vi "LJstreamUD write config.vi"(0 "Working Directory":path, 1 "Data File Prefix":string="data", 2 "Scan Rate (Hz)":dbl=500.0 format="%.3f", 3 "Graph History":i32=1000 min=0, 4 "# Channels":i32=4, 5 "filename":string="ljstreamud.cfg", 6 "Disable Scaling":bool, 7 "Max File Size (Bytes)":i32=1048576, 9 "Write To File":bool, 10 "Channel Setup":T1={"+Ch"=["0", "1", "2", "3", "4", "5", "6", "7"], "-Ch"=["199", "199", "199", "199", "199", "199", "199", "199"], "Ranges"=[0, 0, 0, 0, 0, 0, 0, 0], "Scaling Equation"=["y=v0", "y=v1", "y=v2", "y=v3", "y=v4", "y=v5", "y=v6", "y=v7"], "Graph?"=[]} {"Ranges" items=["LJ_rgBIP10V", "LJ_rgBIP5V", "LJ_rgUNI5V", "LJ_rgUNI2P5V", "LJ_rgUNI1P25V", "LJ_rgBIP1V", "LJ_rgUNIP625V", "LJ_rgBIPP1V", "LJ_rgBIPP01V"]}, 12 "Interval (ms)":u32=500, 13 "Resolution":u8, 14 "SettlingFactor":u8) -> (15 "error out":errorcluster)   [LabVIEW 2021]
uses:
  <vilib>/Utility/config.llb/Write Key (String).vi
  <vilib>/Utility/config.llb/Write Key (U32).vi
  <vilib>/Utility/config.llb/Write Key (Double).vi
  <vilib>/Utility/config.llb/Write Key (I32).vi
  <vilib>/Utility/config.llb/Write Key (Boolean).vi
  <vilib>/Utility/config.llb/NI_LVConfig.lvlib
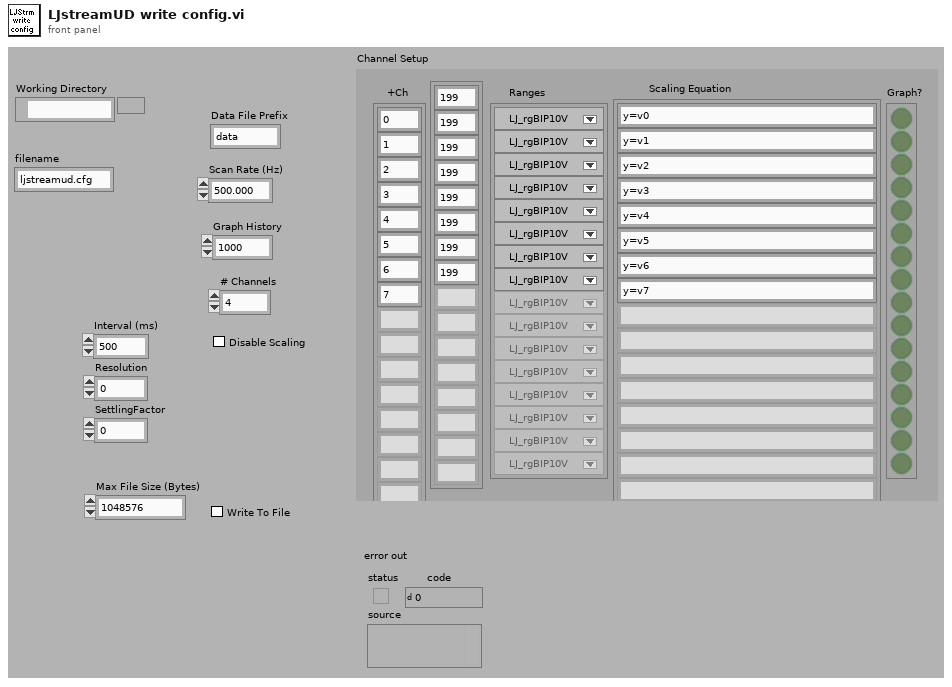
[diagram p1: front panel]
types:
  T1 = cluster{"+Ch":string[], "-Ch":string[], "Ranges":u16[], "Scaling Equation":string[], "Graph?":bool[]}
  T2 = typedef "NI_LVConfig.lvlib/Config Data RefNum.ctl" = refnum<k1>
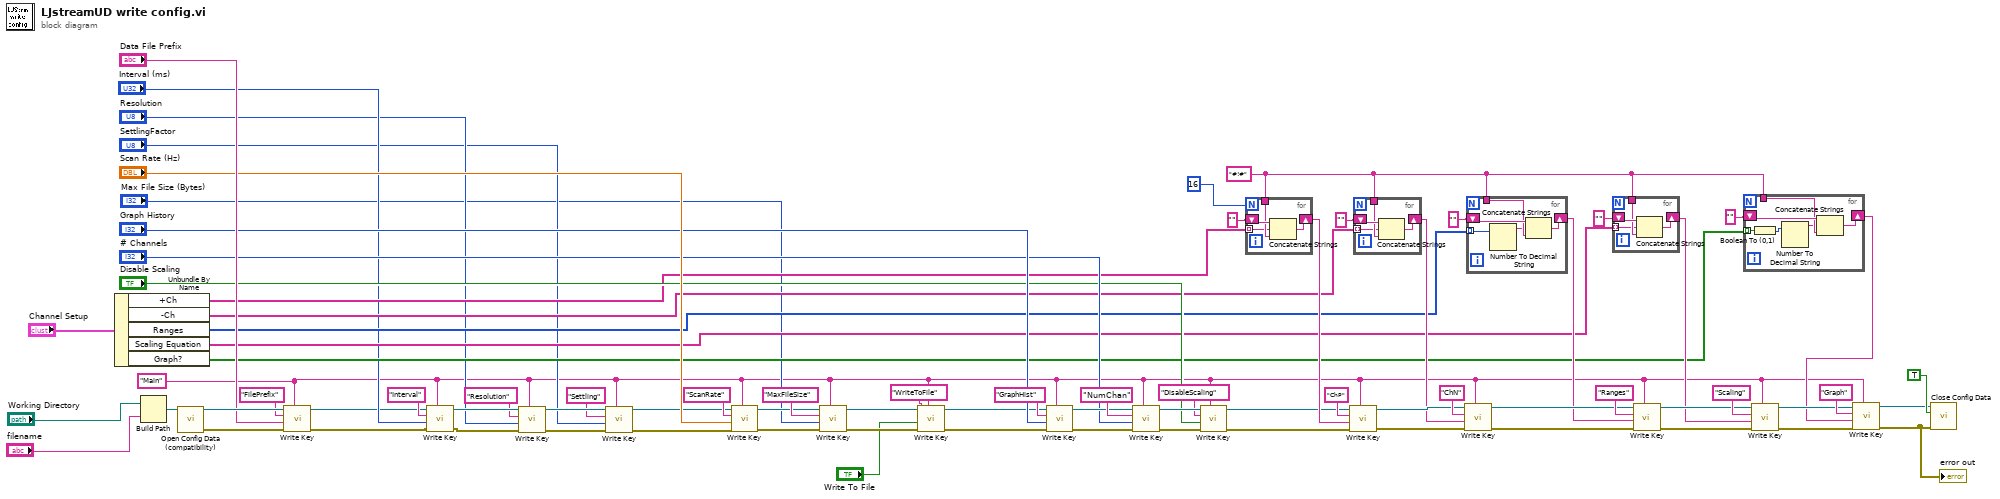
[diagram p0: block diagram]
diagram:
  w43 = "#!#" ("delimiter (Tab)")
  w6 = "Main" ("section")
  n1 = Unbundle By Name("Channel Setup") -> ("+Ch"=w27:string[], "-Ch"=w28:string[], "Ranges"=w29:u16[], "Scaling Equation"=w30:string[], "Graph?"=w31:bool[])
  n2 = Build Path(base path="Working Directory", name or relative path="filename") -> (appended path=w80:path)
  n3 = call <vilib>:"Open Config Data (compatibility).vi"("configuration file path"=w80) -> ("error out"=w78:errorcluster, "refnum"=w79:T2)  [unwired: 8 in, 1 out]
  n4 = call-poly <vilib>:"Write Key.vi"("section"=w6, "error in (no error)"=w78, "value"="Data File Prefix", "key"="FilePrefix", "refnum"=w79) -> ("error out"=w15:errorcluster, "refnum out"=w16:T2)  [unwired: 4 in, 1 out]
  n5 = call-poly <vilib>:"Write Key.vi"("section"=w6, "error in (no error)"=w15, "value"="Interval (ms)", "key"="Interval", "refnum"=w16) -> ("error out"=w24:errorcluster, "refnum out"=w23:T2)  [unwired: 4 in, 1 out]
  n6 = call-poly <vilib>:"Write Key.vi"("section"=w6, "error in (no error)"=w24, "value"="Resolution", "key"="Resolution", "refnum"=w23) -> ("error out"=w26:errorcluster, "refnum out"=w25:T2)  [unwired: 4 in, 1 out]
  n7 = call-poly <vilib>:"Write Key.vi"("section"=w6, "error in (no error)"=w26, "value"="SettlingFactor", "key"="Settling", "refnum"=w25) -> ("error out"=w13:errorcluster, "refnum out"=w14:T2)  [unwired: 4 in, 1 out]
  n8 = call-poly <vilib>:"Write Key.vi"("section"=w6, "error in (no error)"=w13, "value"="Scan Rate (Hz)", "key"="ScanRate", "refnum"=w14) -> ("error out"=w10:errorcluster, "refnum out"=w9:T2)  [unwired: 4 in, 1 out]
  n9 = call-poly <vilib>:"Write Key.vi"("section"=w6, "error in (no error)"=w10, "value"="Max File Size (Bytes)", "key"="MaxFileSize", "refnum"=w9) -> ("error out"=w4:errorcluster, "refnum out"=w5:T2)  [unwired: 4 in, 1 out]
  n10 = call-poly <vilib>:"Write Key.vi"("section"=w6, "error in (no error)"=w4, "value"="Write To File", "key"="WriteToFile", "refnum"=w5) -> ("error out"=w2:errorcluster, "refnum out"=w3:T2)  [unwired: 4 in, 1 out]
  n11 = call-poly <vilib>:"Write Key.vi"("section"=w6, "error in (no error)"=w2, "value"="Graph History", "key"="GraphHist", "refnum"=w3) -> ("error out"=w73:errorcluster, "refnum out"=w74:T2)  [unwired: 4 in, 1 out]
  n12 = call-poly <vilib>:"Write Key.vi"("section"=w6, "error in (no error)"=w73, "value"="# Channels", "key"="NumChan", "refnum"=w74) -> ("error out"=w51:errorcluster, "refnum out"=w52:T2)  [unwired: 4 in, 1 out]
  n13 = call-poly <vilib>:"Write Key.vi"("section"=w6, "error in (no error)"=w51, "value"="Disable Scaling", "key"="DisableScaling", "refnum"=w52) -> ("error out"=w50:errorcluster, "refnum out"=w49:T2)  [unwired: 4 in, 1 out]
  n14 = for {
    N: 16 -> [_]
    shift-right: [w83] -> w56
    shift-left: "" -> [w84]
    tunnel: w43 -> [w82]
    tunnel: w27 -> [w81] mode=indexing
    n15 = Concatenate Strings(w84, w81, w82) -> (w83:string)
  }
  n16 = call-poly <vilib>:"Write Key.vi"("section"=w6, "error in (no error)"=w50, "value"=w56, "key"="ChP", "refnum"=w49) -> ("error out"=w68:errorcluster, "refnum out"=w69:T2)  [unwired: 4 in, 1 out]
  n17 = for {
    shift-right: [w87] -> w55
    shift-left: "" -> [w88]
    tunnel: w43 -> [w86]
    tunnel: w28 -> [w85] mode=indexing
    n18 = Concatenate Strings(w88, w85, w86) -> (w87:string)
  }
  n19 = call-poly <vilib>:"Write Key.vi"("section"=w6, "error in (no error)"=w68, "value"=w55, "key"="ChN", "refnum"=w69) -> ("error out"=w67:errorcluster, "refnum out"=w66:T2)  [unwired: 4 in, 1 out]
  n20 = for {
    shift-right: [w92] -> w54
    shift-left: "" -> [w93]
    tunnel: w43 -> [w91]
    tunnel: w29 -> [w90] mode=indexing
    n21 = Number To Decimal String(number=w90) -> (decimal integer string=w89:string)  [unwired: 1 in]
    n22 = Concatenate Strings(w93, w89, w91) -> (w92:string)
  }
  n23 = for {
    shift-right: [w96] -> w53
    shift-left: "" -> [w97]
    tunnel: w43 -> [w95]
    tunnel: w30 -> [w94] mode=indexing
    n24 = Concatenate Strings(w97, w94, w95) -> (w96:string)
  }
  n25 = call-poly <vilib>:"Write Key.vi"("section"=w6, "error in (no error)"=w67, "value"=w54, "key"="Ranges", "refnum"=w66) -> ("error out"=w64:errorcluster, "refnum out"=w63:T2)  [unwired: 4 in, 1 out]
  n26 = for {
    shift-right: [w102] -> w42
    shift-left: "" -> [w103]
    tunnel: w43 -> [w101]
    tunnel: w31 -> [w98] mode=indexing
    n27 = Boolean To (0,1)(Boolean=w98) -> (0, 1=w99:i16)
    n28 = Number To Decimal String(number=w99) -> (decimal integer string=w100:string)  [unwired: 1 in]
    n29 = Concatenate Strings(w103, w100, w101) -> (w102:string)
  }
  n30 = call-poly <vilib>:"Write Key.vi"("section"=w6, "error in (no error)"=w64, "value"=w53, "key"="Scaling", "refnum"=w63) -> ("error out"=w45:errorcluster, "refnum out"=w44:T2)  [unwired: 4 in, 1 out]
  n31 = call-poly <vilib>:"Write Key.vi"("section"=w6, "error in (no error)"=w45, "value"=w42, "key"="Graph", "refnum"=w44) -> ("error out"=w32:errorcluster, "refnum out"=w41:T2)  [unwired: 4 in, 1 out]
  "error out" <- w32
  n32 = call <vilib>:"Close Config Data.vi"("error in (no error)"=w32, "write file if changed (T)"=TRUE ("write configuration file? (F)"), "refnum"=w41) -> ()  [unwired: 7 in, 2 out]
